vi "Query Power Measurement Elapsed Intervals.vi"(8 "error in (no error)":errorcluster, 9 "Instance (1)":i32=1, 11 "VISA resource name":refnum<visa-resource-name>) -> (0 "error out":errorcluster, 2 "Elapsed Intervals":string, 3 "VISA resource name out":refnum<visa-resource-name>)   [LabVIEW 2020, in "Rohde&Schwarz CMXP GPRF.lvlib"]
doc: "Returns the reliability indicator and the number of elapsed measurement intervals.\n\nAttribute:\nRSCMXPGPRF_ATTR_POWER_MEASUREMENT_ELAPSED_INTERVALS\n\nRemote-control command:\nFETCh:GPRF:MEAS<i>:POWer:ESTatistics?"
uses:
  <instrlib>/Rohde&Schwarz CMXP GPRF/Rohde&Schwarz CMXP GPRF.lvlib
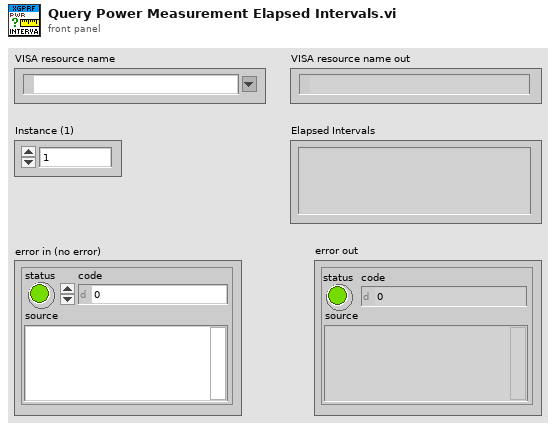
[diagram p1: front panel]
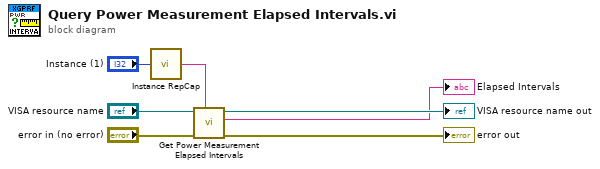
[diagram p0: block diagram]
diagram:
  n1 = call <instrlib>:"Instance RepCap.vi"("Instance in"="Instance (1)") -> ("Instance out"=w2:string)
  n2 = call "Get Power Measurement Elapsed Intervals"("Repeated Capabilities"=w2, "error in (no error)"="error in (no error)", "instrument handle"="VISA resource name") -> ("error out"=→"error out":errorcluster, "Power Measurement Elapsed Intervals"=→"Elapsed Intervals":string, "instrument handle out"=→"VISA resource name out":refnum<visa-resource-name>)  [unwired: 6 in]
